vi "Multiscale Analysis.vi"() -> ()   [LabVIEW 2023]
doc: "This example shows the application of the wavelet transforms in multiscale signal analysis.\n\nThe wavelet-transform based method represents a signal in multiple resolutions. You can learn the global profile as well as the detail of a signal. \n\nThis example uses the WA Discrete Wavelet Transform VI and the Inverse Discrete Wavelet Transform VI to perform multiscale analysis on a Standard & Poor's (S&P) stock index record. \n\n<b>Instructions:</b>\n1) Run this VI.\n2) Observe the short-term, medium-term and long-term variation of the signal."
uses:
  <vilib>/addons/Wavelet Analysis/discrete wavelet transform.llb/WA 1D Discrete Wavelet Transform (Array).vi
  <vilib>/addons/_Advanced Signal Processing/NI_AdvSigProcWA.lvlib
panel:
  in  "Data":u16(ring)=107 items=["Doppler"=102, "HOP"=103, "TF Sine"=104, "Noisy Doppler"=105, "Sea Temperature"=106, "Sp500"=107, "Power Line"=108, "Engine Knocking"=109, "HeaviSine"=110, "Bumps"=111, "Blocks"=112, "Piece Regular"=113, "HypChirps"=114, "LinChirps"=115, "Chirps"=116, "Piece Polynomial"=117, "ECG"=131]
  out "Long-Term Trend":dbl[](graph)
  out "Medium-Term Variation":dbl[](graph)
  out "Short-Term Variation":dbl[](graph)
  out "Signal":dbl[](graph)
  in  "Wavelet":u16(ring) items=["db02"=0, "db03"=1, "db04"=2, "db05"=3, "db06"=4, "db07"=5, "db08"=6, "db09"=7, "db10"=8, "db11"=9, "db12"=10, "db13"=11, "db14"=12, "Haar"=13, "bior1_3"=14, "bior1_5"=15, "bior2_2"=16, "bior2_4"=17, "bior2_6"=18, "bior2_8"=19, "bior3_1"=20, "bior3_3"=21, "bior3_5"=22, "bior3_7"=23, "bior3_9"=24, "bior4_4 (FBI)"=25, "bior5_5"=38, "bior6_8"=39, "coif1"=26, "coif2"=27, "coif3"=28, "coif4"=29, "coif5"=30, "sym2"=31, "sym3"=32, "sym4"=33, "sym5"=34, "sym6"=35, "sym7"=36, "sym8"=37]
  in  "stop":bool
  # "Overview: Shows the application of the wavelet transforms in multiscale signal analysis.\nRequirements: LabVIEW Full Development System, Advanced Signal Processing Toolkit\nInstructions: \n1. Run this VI.\n2. Observe the short-term, medium-term and long-term variation of the signal.\n3. Click Stop to stop the VI."
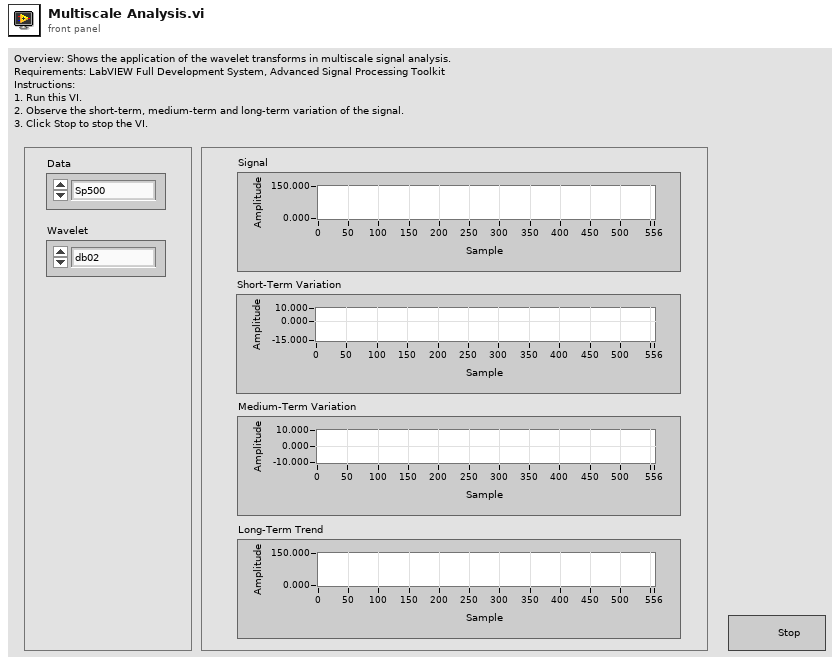
[diagram p1: front panel]
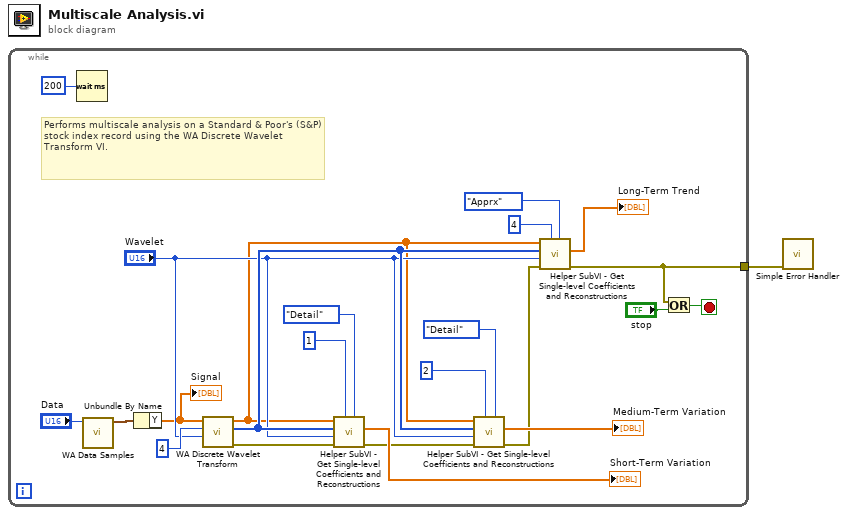
[diagram p0: block diagram]
diagram:
  n1 = while {
    tunnel: [w2] -> w1
    stop <- w24 stop-if-true
    # "Performs multiscale analysis on a Standard & Poor's (S&P) stock index record using the WA Discrete Wavelet Transform VI."
    n2 = Wait (ms)(milliseconds to wait=u32 200 ("millisecond multiple")) -> ()  [unwired: 1 out]
    n3 = call <vilib>:"WA Data Samples.vi"("data"="Data") -> ("signal"=w22:waveform(dbl))  [unwired: 10 out]
    n4 = Unbundle By Name(w22) -> ("Y"=w10:dbl[])
    "Signal" <- w10
    n5 = call-poly <vilib>:"WA Discrete Wavelet Transform.vi"("wavelet"="Wavelet", "levels"=4, "signal"=w10) -> ("error out"=w20:errorcluster, "length"=w13:i32[], "DWT coef"=w11:dbl[])  [unwired: 1 in, 5 out]
    n6 = call "Helper SubVI - Get Single-level Coefficients and Reconstructions.vi"("type"=enum16{"Apprx", "Detail"}."Detail", "level"=1, "error in (no error)"=w20, "wavelet"="Wavelet", "Lengths"=w13, "DWT"=w11) -> ("error out"=w5:errorcluster, "Reconstruction"=→"Short-Term Variation":dbl[])  [unwired: 3 in, 1 out]
    n7 = call "Helper SubVI - Get Single-level Coefficients and Reconstructions.vi"("type"=enum16{"Apprx", "Detail"}."Detail", "level"=2 ("level 2"), "error in (no error)"=w5, "wavelet"="Wavelet", "Lengths"=w13, "DWT"=w11) -> ("error out"=w4:errorcluster, "Reconstruction"=→"Medium-Term Variation":dbl[])  [unwired: 3 in, 1 out]
    n8 = call "Helper SubVI - Get Single-level Coefficients and Reconstructions.vi"("type"=enum16{"Apprx", "Detail"}."Apprx", "level"=4 ("level 3"), "error in (no error)"=w4, "wavelet"="Wavelet", "Lengths"=w13, "DWT"=w11) -> ("error out"=w2:errorcluster, "Reconstruction"=→"Long-Term Trend":dbl[])  [unwired: 3 in, 1 out]
    n9 = Or(x=w2, y="stop") -> (x .or. y?=w24:bool)
  }
  n10 = call <vilib>:"Simple Error Handler.vi"("error in (no error)"=w1) -> ()  [unwired: 1 in, 8 out]
